vi "FindT_totune_to.vi"(9 "T from":dbl=53.0) -> (3 "T2 tune to":dbl=97.72219547120214)   [LabVIEW 2010]
uses:
  <vilib>/gmath/NI_Gmath.lvlib
panel:
  in  "T to tune to":dbl=53.0
  out "Temperature vs refractive index":cluster{"Refr index raw":dbl[], "yi":dbl[]}[](graph)=[{"Refr index raw"=[3.51113, 3.51123, 3.51146, 3.51181, 3.51229, 3.51288, 3.51358, 3.51439, 3.51979, 3.52703, 3.53555, 3.54394], "yi"=[30.0, 40.0, 50.0, 60.0, 70.0, 80.0, 90.0, 100.0, 150.0, 200.0, 250.0, 295.0]}, {"Refr index raw"=[3.514190063648601], "yi"=[97.72219547120214]}]
  in  "method":i32(ring)=3 items=["nearest", "linear", "spline", "cubic Hermite", "Lagrange"]
  out "Silicon refr index at Tslave":dbl[](array[numeric])=[97.72219547120214]
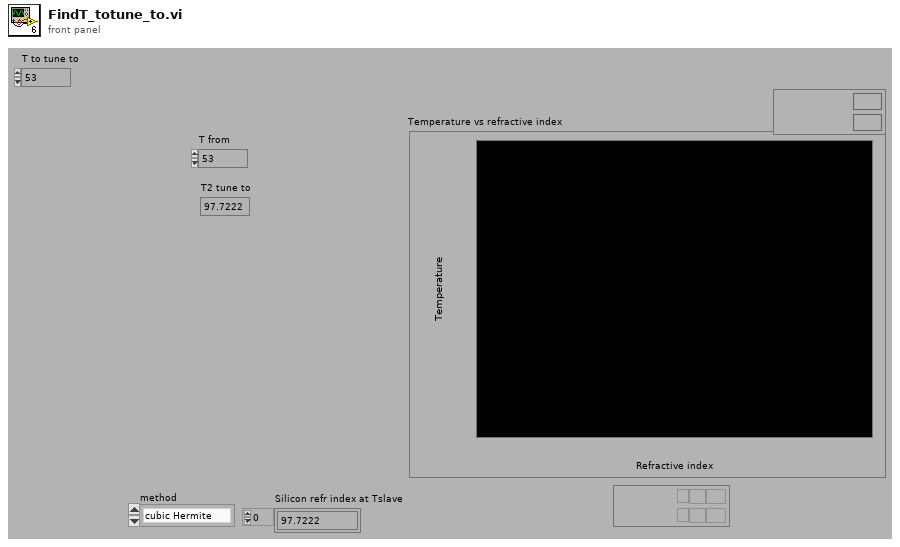
[diagram p1: front panel]
types:
  T1 = cluster{"Silicon refr index at T":dbl[], "f":dbl[]}
  T2 = cluster{"Silicon refr index at T":dbl[], "f":dbl[]}[]
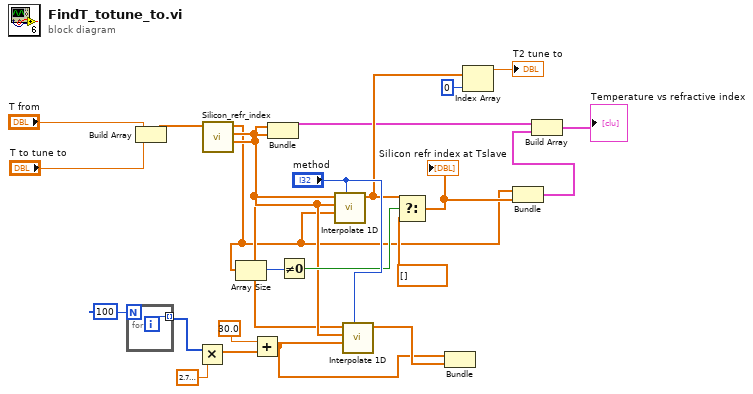
[diagram p0: block diagram]
diagram:
  n1 = for {
    N: 100 -> [_]
    tunnel: [w25] -> w22 mode=indexing
    i -> [w25]
  }
  n2 = Build Array("T from", "T to tune to") -> (w4:dbl[])
  n3 = Multiply(x=w22, y=sgl 2.7) -> (x*y=w20:sgl[])
  n4 = call "Silicon_refr_index.vi"("Temperature"=w4) -> ("Refr index raw"=w11:dbl[], "T raw"=w5:dbl[], "Silicon refr index at T"=w1:dbl[])  [unwired: 8 in]
  n5 = Array Size(array=w1) -> (size(s)=w14:i32)
  n6 = Add(x=sgl 30.0, y=w20) -> (x+y=w16:sgl[])
  n7 = Bundle("Refr index raw"=w11, "T raw"=w5) -> (w8:cluster{"Refr index raw":dbl[], "T raw":dbl[]})  [unwired: 1 in]
  n8 = Not Equal To 0?(x=w14) -> (x != 0?=w13:bool)
  n9 = call <vilib>:"Interpolate 1D.vi"("method"="method", "xi"=w1, "X"=w11, "Y"=w5) -> ("yi"=w10:dbl[])  [unwired: 5 in, 2 out]
  n10 = call <vilib>:"Interpolate 1D.vi"("method"="method", "xi"=w16, "X"=w11, "Y"=w5) -> ("yi"=w17:dbl[])  [unwired: 5 in, 2 out]
  n11 = Select(t=w10, s=w13, f=dbl[] []) -> (s? t:f=w15:dbl[])
  "Silicon refr index at Tslave" <- w15
  n12 = Bundle(w16, "yi"=w17) -> ()  [unwired: 1 in, 1 out]
  n13 = Index Array(array=w10, index=0) -> (element=→"T2 tune to":dbl)
  n14 = Bundle("Silicon refr index at T"=w1, "f"=w15) -> (w7:T1)  [unwired: 1 in]
  n15 = Build Array(w8, w7) -> (→"Temperature vs refractive index":T2)
